vi "Globals.vi"() -> ()   [LabVIEW 2012]
uses:
  C:/Program Files/LeddarTech/xtec/LeddarNET2.dll
panel:
  in  "New Status":bool
  in  "Detections":refnum<k24>[](array[refnum])
  # "Global variables used to transfer data from\nthe DataReceived_CB to the LeddarGetData"
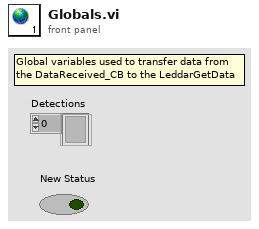
[diagram p1: front panel]
diagram:
